vi "2012_07_10_each motor.vi"(0 "MC Power Data In":waveform(dbl)[](array[waveform]), 1 "Motor Power Data In":waveform(dbl)[](array[waveform]), 5 "Power \nSetting":i8(slide) min=0 max=100 step=10 scale=0.0..100.0, 7 "On/Off Control":T1(ring), 9 "Motor":i16=1, 11 "Error In":errorcluster, 12 "Fine Data In":dbl[][][](array[numeric])) -> (6 "Power \nSetting":i8(slide) min=0 max=100 step=10 scale=0.0..100.0, 14 "Fine Data Out":dbl[][][](array[numeric]), 15 "Errors":errorcluster)   [LabVIEW 2011]
uses:
  <vilib>/express/express arith-compare/Formula/XNode/ExpressFormulaBlockNode.xnode
  <vilib>/Analysis/NI_AALBase.lvlib
panel:
  out "Efficiency (%)":dbl format="%#.4f"
  in  "Manual Save\nFine Event":bool
  in  "Motor1 ID":string
  in  "User":string
  in  "Comments (cleared when written to file)":string
  out "Elapsed Time (s)":string caption="Elapsed Time Text"
  out "Start Time":string caption="Start Time Text"
  in  "Motor Failure\n(Click to clear)":bool
  out "Coarse":bool caption="Time has Elapsed"
  out "Fine":bool caption="Time has Elapsed"
  out "Temps":dynamicdata(graph) caption="Signal Out"
  out "Power Graph":dynamicdata(graph) caption="Collected Signals"
  out "RPM":dynamicdata(graph) caption="Collected Signals"
  out "Motor RPM":dbl format="%#.0f"
  out "Power to Motor (W)":dbl format="%#.4f"
  out "Power to MC (W)":dbl format="%#.4f"
  out "Supply Voltage (V)":dbl format="%#.4f"
  in  "Run":bool
  out "Motor Temp (F)":dbl format="%.1f"
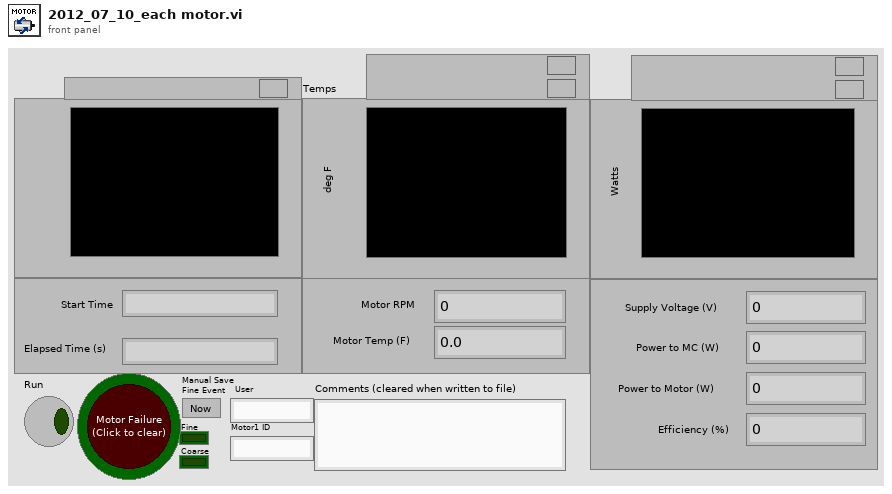
[diagram p1: front panel]
types:
  T1 = enum8{"Enabled", "Disabled", "Disabled and Grayed Out"}
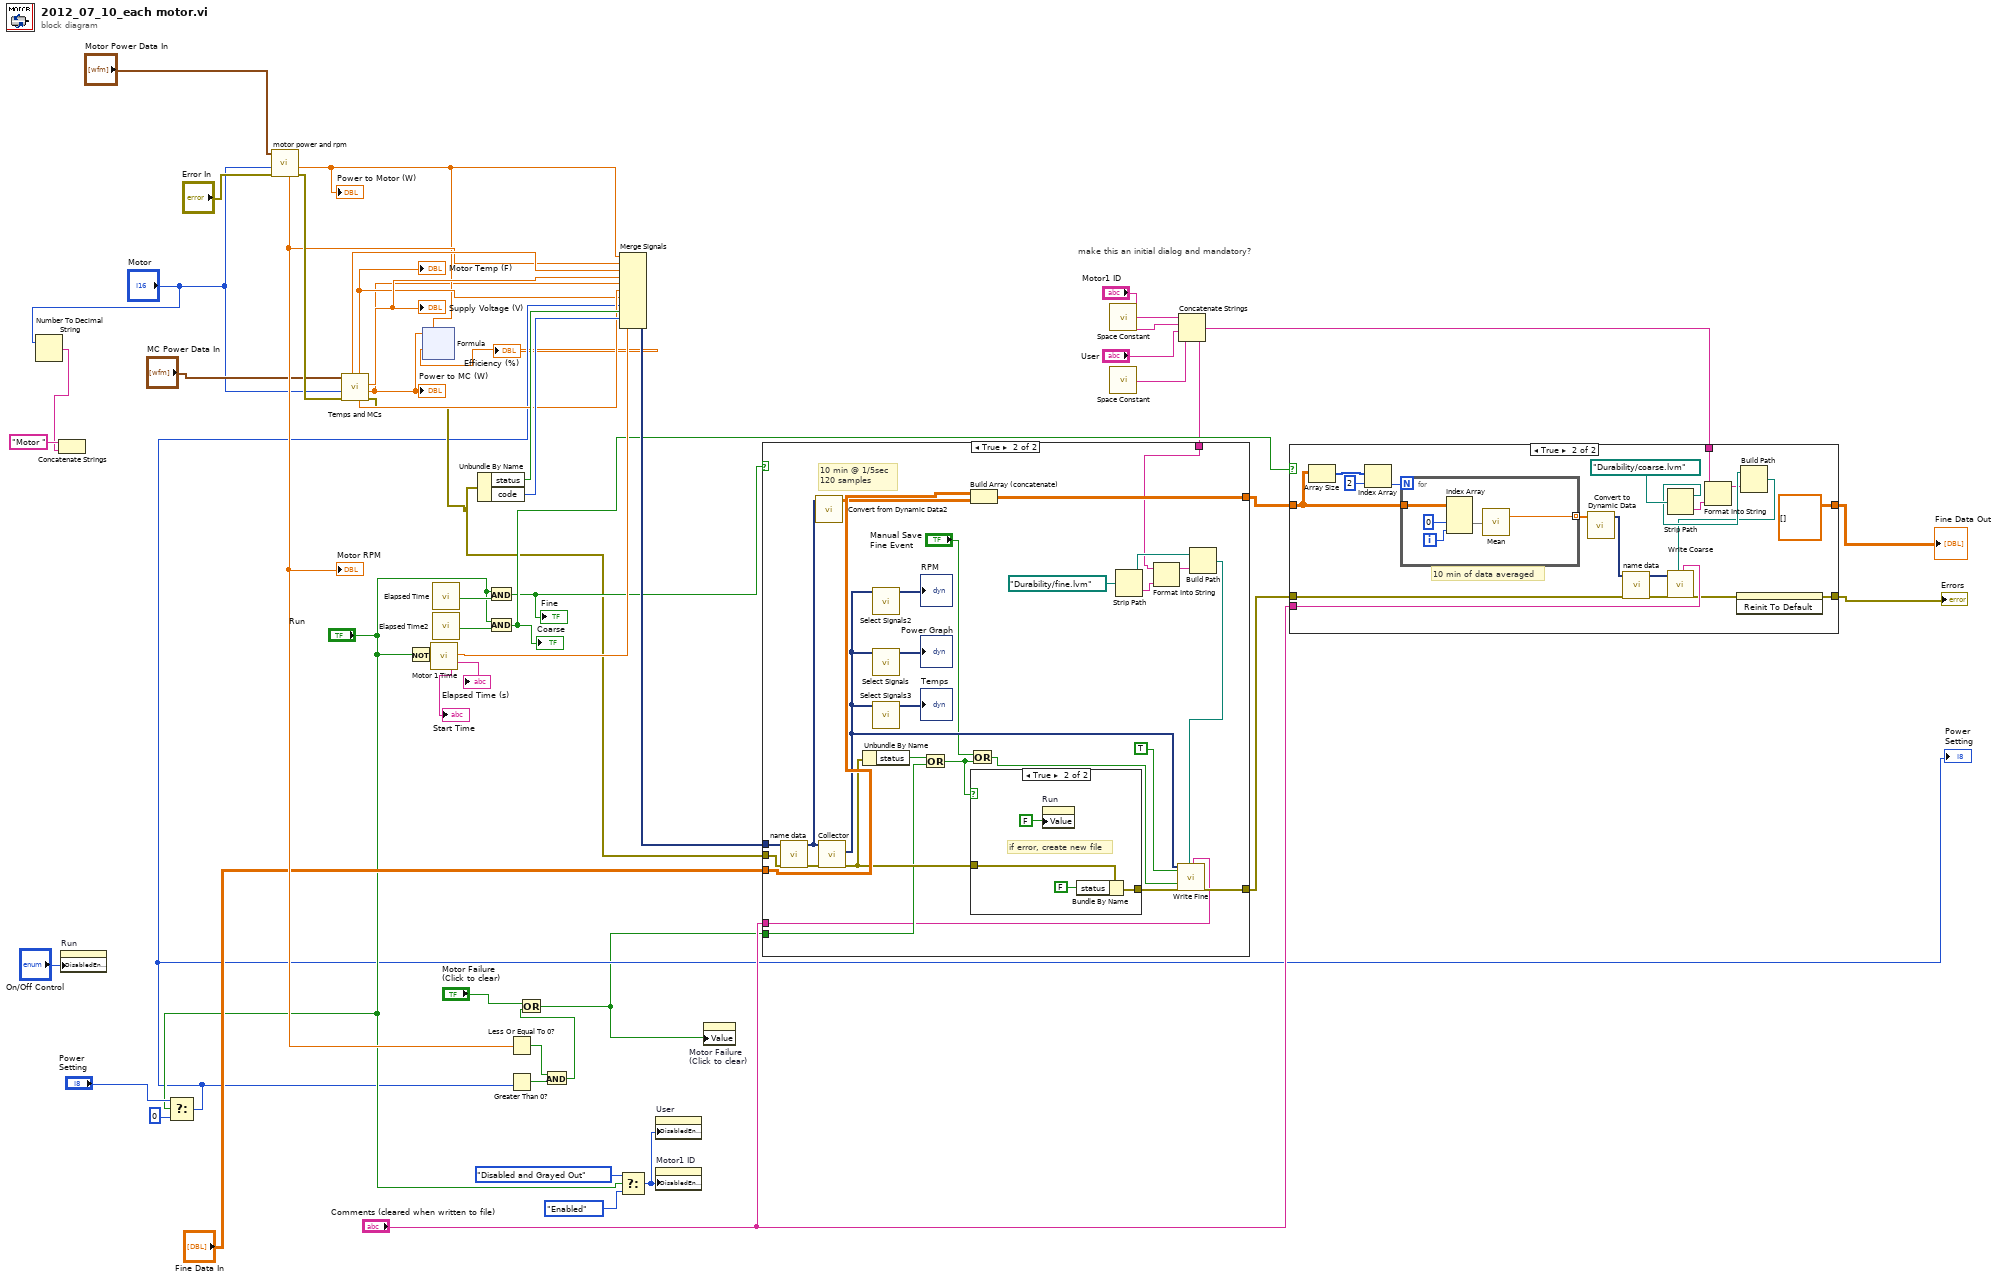
[diagram p0: block diagram]
diagram:
  # "make this an initial dialog and mandatory?"
  n1 = Number To Decimal String(number="Motor") -> (decimal integer string=w6:string)  [unwired: 1 in]
  n2 = Concatenate Strings("Motor ", w6) -> ()  [unwired: 1 out]
  n3 = property on="Run" class="Bool (strict)"("DisabledEnum"="On/Off Control") -> ()  [unwired: 2 in, 2 out]
  n4 = Select(t="Power \nSetting", s="Run", f=i8 0) -> (s? t:f=w9:i8)
  "Power \nSetting" <- w9
  n5 = call "motor power and rpm.vi"("error in (no error)"="Error In", "Motor"="Motor", "data"="Motor Power Data In") -> ("error out"=w51:errorcluster, "DC value"=w26:dbl, "Numeric"=w40:dbl)  [unwired: 4 in, 2 out]
  "Motor RPM" <- w40
  "Power to Motor (W)" <- w26
  n6 = call "Temps and MCs.vi"("error in (no error)"=w51, "Motor"="Motor", "data"="MC Power Data In") -> ("error out"=w13:errorcluster, "Numeric"=w25:dbl, "DC value 3"=w46:dbl, "DC value 2"=w45:dbl, "DC value"=w44:dbl, "Numeric 2"=w50:dbl)  [unwired: 3 in]
  "Motor Temp (F)" <- w44
  "Supply Voltage (V)" <- w46
  "Power to MC (W)" <- w25
  n7 = Not(x="Run") -> (.not. x?=w35:bool)
  n8 = xnode ("Formula")("MC PWR"=w25, "M PWR"=w26) -> ("Result"=→"Efficiency (%)":dbl)  [unwired: 1 in, 1 out]
  n9 = call "Motor 1 Time"("Reset"=w35) -> ("Start Time Text"=→"Start Time":string, "Elapsed Time (s)"=w34:dbl, "Elapsed Time Text"=→"Elapsed Time (s)":string)  [unwired: 11 in, 5 out]
  n10 = call "Elapsed Time"() -> ("Time has Elapsed"=w27:bool)  [unwired: 12 in, 7 out]
  n11 = call "Elapsed Time2"() -> ("Time has Elapsed"=w30:bool)  [unwired: 12 in, 7 out]
  n12 = Unbundle By Name(w13) -> ("status"=w49:bool, "code"=w48:i32)
  n13 = And(x="Run", y=w27) -> (x .and. y?=w28:bool)
  "Fine" <- w28
  n14 = And(x="Run", y=w30) -> (x .and. y?=w29:bool)
  "Coarse" <- w29
  n15 = Less Or Equal To 0?(x=w40) -> (x <= 0?=w39:bool)
  n16 = Greater Than 0?(x=w9) -> (x > 0?=w38:bool)
  n17 = And(x=w39, y=w38) -> (x .and. y?=w3:bool)
  n18 = Or(x="Motor Failure\n(Click to clear)", y=w3) -> (x .or. y?=w1:bool)
  n19 = Merge Signals(w26, w40, w50, w46, w25, w45, w44, w9, w49, w48, w34) -> (w47:dynamicdata)
  n20 = Select(t=T1."Disabled and Grayed Out" ("Disabled"), s="Run", f=T1."Enabled" ("Disabled")) -> (s? t:f=w31:T1)
  n21 = property on="User" class="Str"("DisabledEnum"=w31) -> ()  [unwired: 2 in, 2 out]
  n22 = property on="Motor1 ID" class="Str"("DisabledEnum"=w31) -> ()  [unwired: 2 in, 2 out]
  n23 = property on="Motor Failure\n(Click to clear)" class="Bool (strict)"("Value"=w1) -> ()  [unwired: 2 in, 2 out]
  n24 = call <vilib>:"Space Constant.vi"() -> ("String"=w19:string)
  n25 = call <vilib>:"Space Constant.vi"() -> ("String"=w17:string)
  n26 = Concatenate Strings("Motor1 ID", w19, "User", w17) -> (w16:string)
  n27 = case shown="True" w28 {
    tunnel: w47 -> [_ w76]
    tunnel: w13 -> [w53 w73]
    tunnel: [w53 w68] -> w41
    tunnel: [w52 w80] -> w42
    tunnel: "Fine Data In" -> [w52 w79]
    tunnel: w1 -> [_ w64]
    tunnel: "Comments (cleared when written to file)" -> [_ w63]
    tunnel: w16 -> [_ w55]
    frame False {
    }
    frame True {
      # "10 min @ 1/5sec\n120 samples"
      n28 = call "name data.vi"("error in (no error)"=w73, "Dynamic Data"=w76) -> ("error out"=w74:errorcluster, "Output"=w75:dynamicdata)  [unwired: 8 in]
      n29 = call "Convert from Dynamic Data2"("Dynamic Data Type"=w75) -> ("Array"=w78:dbl[][])  [unwired: 3 in]
      n30 = call "Collector"("error in (no error)"=w74, "Signals"=w75) -> ("error out"=w66:errorcluster, "Collected Signals"=w69:dynamicdata)  [unwired: 8 in]
      n31 = Unbundle By Name(w66) -> ("status"=w65:bool)
      n32 = call "Select Signals2"("Signals"=w69) -> ("Signal Out"=→"RPM":dynamicdata)  [unwired: 9 in, 1 out]
      n33 = call "Select Signals"("Signals"=w69) -> ("Signal Out"=→"Power Graph":dynamicdata)  [unwired: 9 in, 1 out]
      n34 = call "Select Signals3"("Signals"=w69) -> ("Signal Out"=→"Temps":dynamicdata)  [unwired: 9 in, 1 out]
      n35 = Or(x=w65, y=w64) -> (x .or. y?=w62:bool)
      n36 = Or(x="Manual Save\nFine Event", y=w62) -> (x .or. y?=w61:bool)
      n37 = Build Array (concatenate)(w79, w78) -> (w80:dbl[][][])
      n38 = case shown="True" w62 {
        tunnel: [w81 w85] -> w67
        tunnel: w66 -> [w81 w84]
        frame False {
        }
        frame True {
          # "if error, create new file"
          n39 = property on="Run" class="Bool (strict)"("Value"=FALSE ("Manual Start")) -> ()  [unwired: 2 in, 2 out]
          n40 = Bundle By Name(cluster=w84, "status"=FALSE) -> (w85:errorcluster)
        }
      }
      n41 = Strip Path(path=path "Durability/fine.lvm" ("Filename")) -> (stripped path=w58:path, name=w54:string)
      n42 = Format Into String(initial string=w55, w54) -> (resulting string=w59:string)  [unwired: 2 in, 1 out]
      n43 = Build Path(base path=w58, name or relative path=w59) -> (appended path=w56:path)
      n44 = call "Write Fine"("Signals"=w69, "Reset"=TRUE, "new_file"=w61, "error in (no error)"=w67, "Filename"=w56, "Comment"=w63) -> ("error out"=w68:errorcluster)  [unwired: 11 in, 2 out]
    }
  }
  n45 = case shown="True" w29 {
    tunnel: w42 -> [w87 w106]
    tunnel: [w87 dbl[][][] []] -> w43
    tunnel: w41 -> [w86 w98]
    tunnel: [w86 w94] -> w22
    tunnel: "Comments (cleared when written to file)" -> [_ w96]
    tunnel: w16 -> [_ w89]
    frame False {
    }
    frame True {
      # "10 min of data averaged"
      n46 = Array Size(array=w106) -> (size(s)=w102:i32[])
      n47 = Index Array(array=w102, index=2) -> (element=w103:i32)
      n48 = for {
        N: w103 -> [_]
        tunnel: w106 -> [w111]
        tunnel: [w107] -> w101 mode=indexing
        i -> [w110]
        n49 = Index Array(array=w111, index (dim 1)=0 ("disabled index (row)"), index (dim 2)=w110) -> (element=w109:dbl[])  [unwired: 1 in]
        n50 = call <vilib>:"Mean.vi"("X"=w109) -> ("mean"=w107:dbl)  [unwired: 1 out]
      }
      n51 = call "Convert to Dynamic Data"("Array"=w101) -> ("Dynamic Data Type"=w100:dynamicdata)  [unwired: 3 in]
      n52 = call "name data.vi"("error in (no error)"=w98, "Dynamic Data"=w100) -> ("error out"=w97:errorcluster, "Output"=w99:dynamicdata)  [unwired: 8 in]
      n53 = Strip Path(path=path "Durability/coarse.lvm" ("Filename")) -> (stripped path=w92:path, name=w90:string)
      n54 = Format Into String(initial string=w89, w90) -> (resulting string=w91:string)  [unwired: 2 in, 1 out]
      n55 = Build Path(base path=w92, name or relative path=w91) -> (appended path=w88:path)
      n56 = call "Write Coarse"("Signals"=w99, "error in (no error)"=w97, "Filename"=w88, "Comment"=w96) -> ("error out"=w95:errorcluster)  [unwired: 13 in, 2 out]
      n57 = invoke on="Comments (cleared when written to file)" class="Str" method="Reinit To Default"(error in=w95) -> (error out=w94:errorcluster)  [unwired: 2 in, 2 out]
    }
  }
  "Errors" <- w22
  "Fine Data Out" <- w43
